vi "Interpret Key Down.vi"(9 "Char":i16, 10 "VKey":T1) -> (2 "Enum":T2(ring))   [LabVIEW 2011]
uses:
  <vilib>/event_ctls.llb/eventvkey.ctl
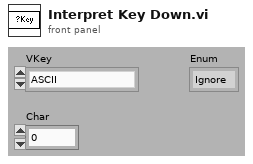
[diagram p1: front panel]
types:
  T1 = typedef "eventvkey.ctl" = enum16{"ASCII", "Enter", "Return", "Shift", "Ctrl", "Alt", "Cmd", "Opt", "Caps", "NumLock", "Clear", "Break", "Up", "Down", "Left", "Right", "Insert", "Delete", "Home", "End", "PageUp", "PageDown", "Escape", "Help", "Pause", "ScrollLock", "F1", "F2", "F3", "F4", "F5", "F6", "F7", "F8", "F9", "F10", "F11", "F12", "F13", "F14", "F15", "F16", "F17", "F18", "F19", "F20", "F21", "F22", "F23", "F24", "Play", "VolumeUp", "VolumeDown", "Mute", "Two Byte Char"}
  T2 = enum16{"Ignore", "Left", "Right", "Up", "Down", "CL", "CC"}
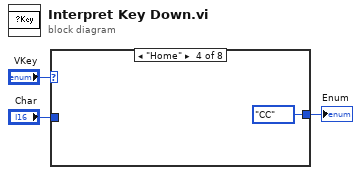
[diagram p0: block diagram]
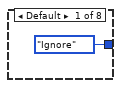
[diagram p2: hidden frame]
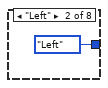
[diagram p3: hidden frame]
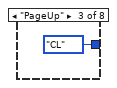
[diagram p4: hidden frame]
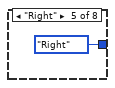
[diagram p5: hidden frame]
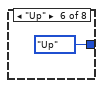
[diagram p6: hidden frame]
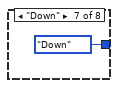
[diagram p7: hidden frame]
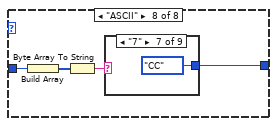
[diagram p8: hidden frame]
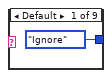
[diagram p9: hidden frame]
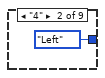
[diagram p10: hidden frame]
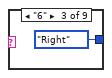
[diagram p11: hidden frame]
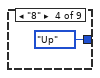
[diagram p12: hidden frame]
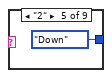
[diagram p13: hidden frame]
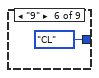
[diagram p14: hidden frame]
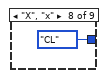
[diagram p15: hidden frame]
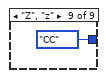
[diagram p16: hidden frame]
diagram:
  n1 = case shown="\"Home\"" "VKey" {
    tunnel: "Char" -> [_ _ _ _ _ _ _ w14]
    tunnel: [T2."Ignore" T2."Left" T2."CL" T2."CC" T2."Right" T2."Up" T2."Down" w11] -> w1
    frame Default {
    }
    frame "Left" {
    }
    frame "PageUp" {
    }
    frame "Home" {
    }
    frame "Right" {
    }
    frame "Up" {
    }
    frame "Down" {
    }
    frame "ASCII" {
      n2 = Build Array(w14) -> (w13:i16[])
      n3 = Byte Array To String(unsigned byte array=w13) -> (string=w12:string)
      n4 = case shown="\"7\"" w12 {
        tunnel: [T2."Ignore" T2."Left" T2."Right" T2."Up" T2."Down" T2."CL" T2."CC" T2."CL" T2."CC"] -> w11
        frame Default {
        }
        frame "4" {
        }
        frame "6" {
        }
        frame "8" {
        }
        frame "2" {
        }
        frame "9" {
        }
        frame "7" {
        }
        frame "X", "x" {
        }
        frame "Z", "z" {
        }
      }
    }
  }
  "Enum" <- w1
